vi "_Update Start Up Turbo.vi"(4 "error in (no error)":errorcluster) -> (0 "error Out":errorcluster, 2 "Next InstrState":T1, 3 "Cancel":bool)   [LabVIEW 2012]
uses:
  Type/_RT Instrument State.ctl
  Type/_LCD Line1 Msg.ctl
  Type/_LCD Line2 Msg.ctl
  Type/_Pump Parameter.ctl
  Type/_RW Status.ctl
  Type/_LED States.ctl
  _RT Global.vi
  <vilib>/Utility/error.llb/Error Cluster From Error Code.vi
  <vilib>/rvi/errors/niLvFpgaAdjustHostInterfaceError.vi
  <vilib>/rvi/interface/nirviReadWriteControl/nirviReadWriteControl.xnode
  FPGA Bitfiles/FPGA9602.lvbitx
  NiFpgaLv.dll
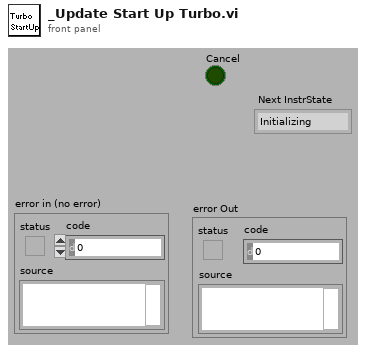
[diagram p1: front panel]
types:
  T1 = typedef "_RT Instrument State.ctl" = enum16{"Initializing", "Mass Spectrometer is Off", "Starting Up", "Turning Power Off", "Going to Standby", "Roughing Pump Ready", "Turning Turbo Off", "Turbo Startup", "Turbopump Ready", "Checking Vacuum", "Going to Ready", "Ready", "Running", "Source Standby", "Lost Communication", "Shutting Down", "Fault", "24V Standby", "Go to 24V Standby", "Turbopump Ready-Waiting"}
  T2 = typedef "_Pump Parameter.ctl" = enum16{"Turn Pump Motor On", "Turn Pump Motor Off", "Read Pump Oil Deficiency", "Read Rotation Switch Point Attained", "Read Ele. Drive Over Temperature", "Read Pump Over Temperature", "Read Set Rotation Speed Attained", "Read Turbopump Accelerates", "Read Actual Rotation Speed in Hz", "Read Motor Current in A", "Read Operating Hours in h", "Read Motor Voltage in V", "Read Motor Power in W", "Set Rotation Speed Switchpoint in %", "Clear Error", "Read Error Code", "Read Bearing Temperature", "Read Hardware Version", "Read Firmware Version", "Read Operating Hours (Drive)", "Read Rotational Speed (rpm)", "Read Power Stage Temperature", "Read Electronics Temperature", "Read Upper Pump Temperature", "Read Motor Temperature", "Read Error Code History, 1", "Read Error Code History, 2", "Read Error Code History, 3", "Read Error Code History, 4", "Read Error Code History, 5", "Read Error Code History, 6", "Read Error Code History, 7", "Read Error Code History, 8", "Read Error Code History, 9", "Read Error Code History, 10"}
  T3 = typedef "_RW Status.ctl" = enum8{"Done", "Do Read", "Do Write", "Set Latch1", "Set Latch2", "Set Latch3", "Set Latch4", "RP ON", "EL ON", "Serial Send", "Set LC Out", "Get LC In", "Read VAC", "Table Test", "Get Interlock", "Do Read2", "Do Write2"}
  T4 = typedef "_LED States.ctl" = enum8{"Idle", "Solid B", "Solid R", "Solid P", "Off B", "Off R", "Off P", "Off BRP", "Off RP", "Flash R&P", "Flash P"}
  T5 = typedef "_LCD Line2 Msg.ctl" = u16
  T6 = typedef "_LCD Line1 Msg.ctl" = u16
  T7 = typedef "_RT Startup Options.ctl" = cluster{"Door":bool, "Curtain":bool, "Pressure":bool, "Turbo":bool, "SysPoll":bool, "GasFlag":bool}
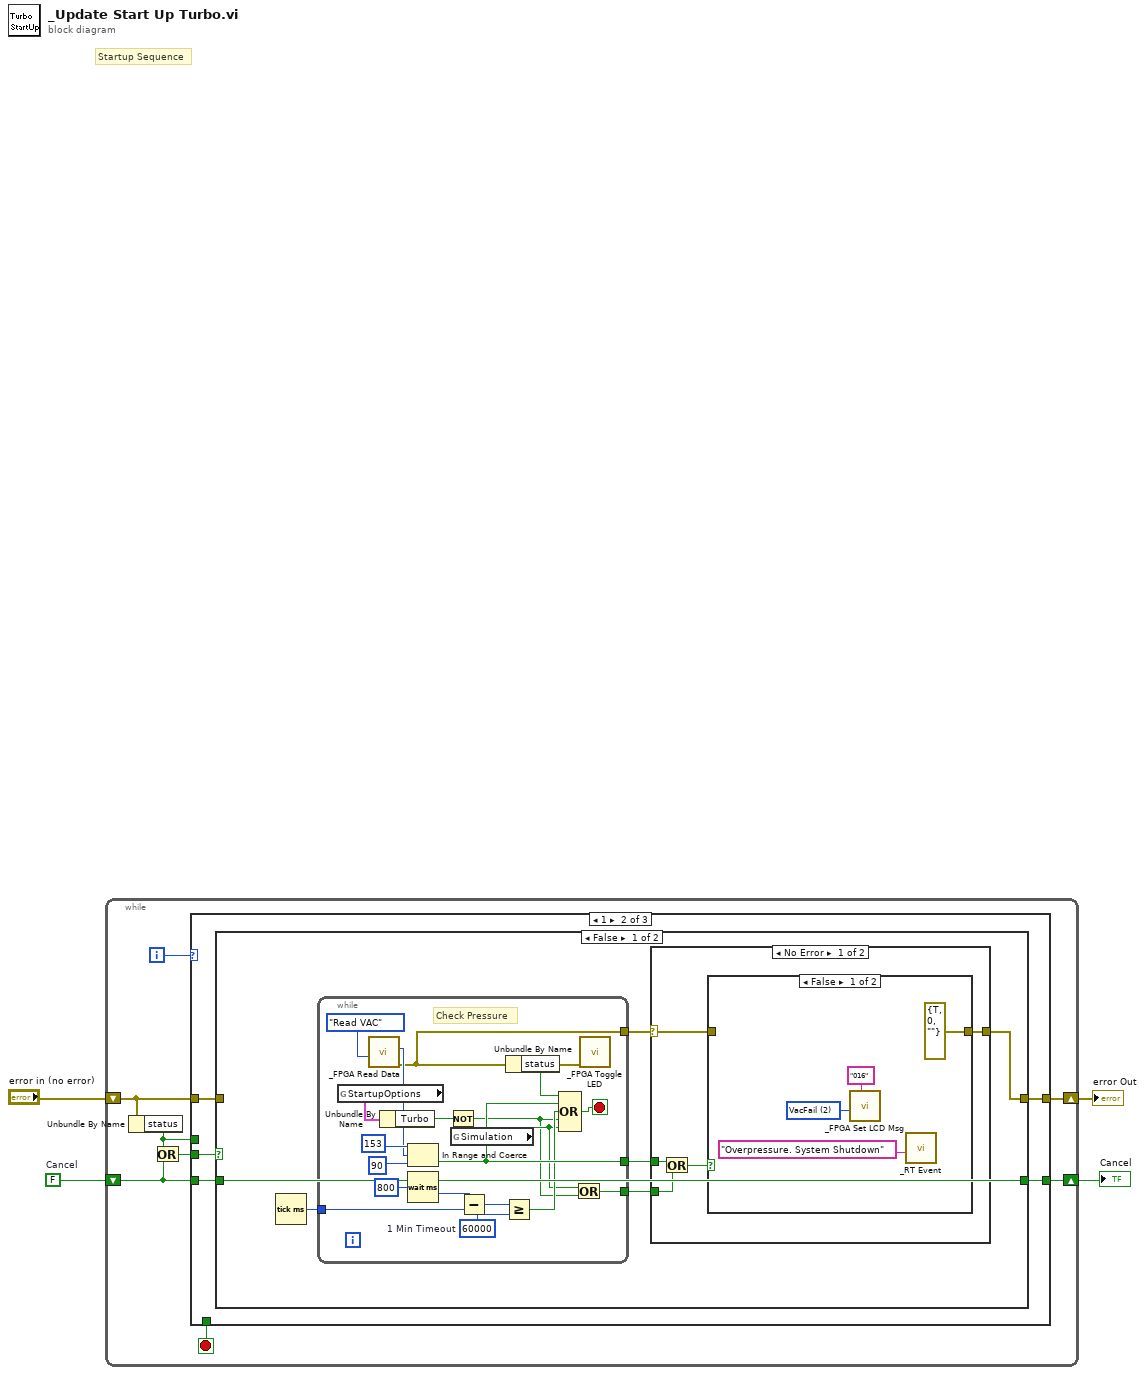
[diagram p0: block diagram]
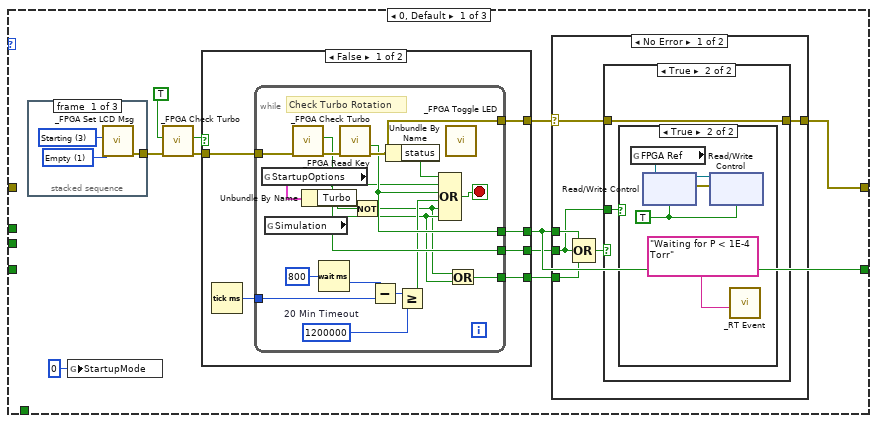
[diagram p2: hidden frame]
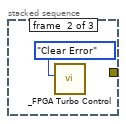
[diagram p3: hidden frame]
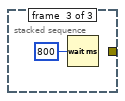
[diagram p4: hidden frame]
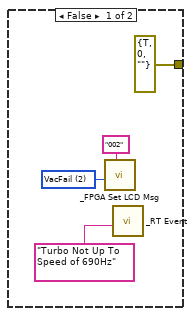
[diagram p6: hidden frame]
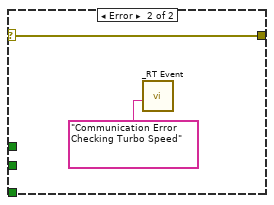
[diagram p8: hidden frame]
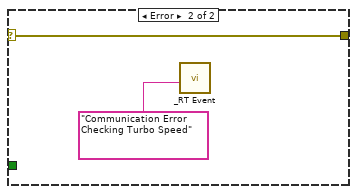
[diagram p10: hidden frame]
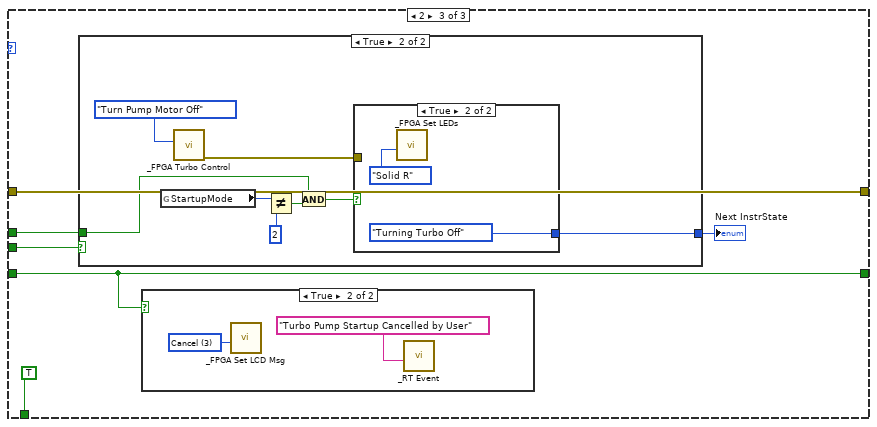
[diagram p12: hidden frame]
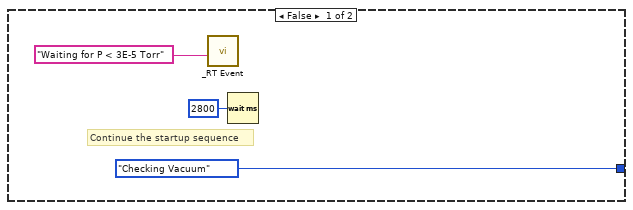
[diagram p13: hidden frame]
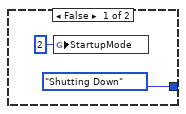
[diagram p14: hidden frame]
diagram:
  w3 = FALSE  # Cancel
  # "Startup Sequence"
  n1 = while {
    shift-right: [w8] -> w2
    shift-left: "error in (no error)" -> [w10]
    shift-right: [w7] -> w1
    shift-left: w3 -> [w9]
    i -> [w12]
    stop <- w6 stop-if-true
    n2 = Unbundle By Name(w10) -> ("status"=w5:bool)
    n3 = Or(x=w5, y=w9) -> (x .or. y?=w11:bool)
    n4 = case shown="1" w12 {
      tunnel: w11 -> [_ w75 w119]
      tunnel: w10 -> [_ w74 w121]
      tunnel: w9 -> [_ w73 w120]
      tunnel: [w22 w77 w121] -> w8
      tunnel: [w21 w76 w120] -> w7
      tunnel: [_ _ TRUE] -> w6
      tunnel: w5 -> [_ _ w117]
      frame 0, Default {
        n5 = stacked-sequence {
          tunnel: [w23 _ _] -> w13
          frame #0 {
            w24 = T5 1 items=["Same", "Empty", "VacFail", "Cancel", "CheckGas", "EleFail", "Probe1Fail", "Probe2Fail", "HeaterFail", "DoorOpen", "CheckComm", "PressStart", "StartRP"] ("Line2Msg (same)")
            w25 = T6 3 items=["Same", "Empty", "Connected", "Starting", "Stopping", "Action", "On", "Service", "Call", "Acquiring", "Source"] ("Line1Msg (same)")
            n6 = call "_FPGA Set LCD Msg.vi"("Line2Msg (same)"=w24, "Line1Msg (same)"=w25) -> ("error out"=w23:errorcluster)  [unwired: 5 in, 2 out]
          }
          frame #1 {
            n7 = call "_FPGA Turbo Control.vi"("Command"=_Pump_Parameter."Clear Error") -> ()  [unwired: 3 in, 6 out]
          }
          frame #2 {
            n8 = Wait (ms)(milliseconds to wait=u32 800) -> ()  [unwired: 1 out]
          }
        }
        n9 = global write "_RT Global.vi" "StartupMode"(u8 0 ("StartupMode")) -> ()
        n10 = call "_FPGA Check Turbo.vi"("error in"=w13, "CheckNow (F)"=TRUE) -> ("error out"=w18:errorcluster, "SpeedOK"=w16:bool)  [unwired: 1 in, 3 out]
        n11 = case shown="False" w16 {
          selector: w16 -> [_ w52]
          tunnel: [w33 _] -> w21
          tunnel: [w32 w53] -> w20
          tunnel: [w31 w52] -> w19
          tunnel: w18 -> [w29 w53]
          tunnel: [w28 _] -> w14
          frame False {
            n12 = Tick Count (ms)() -> (millisecond timer value=w30:u32)
            n13 = while {
              tunnel: w29 -> [w42]
              tunnel: [w48] -> w32
              tunnel: [w47] -> w33
              tunnel: w30 -> [w43]
              tunnel: [w40] -> w31
              tunnel: [w37] -> w28
              stop <- w51 stop-if-true
              w46 = u32 1200000  # 20 Min Timeout
              # "Check Turbo Rotation"
              n14 = global read "_RT Global.vi" "StartupOptions"() -> (w36:T7)
              n15 = global read "_RT Global.vi" "Simulation"() -> (w38:bool)
              n16 = call "_FPGA Check Turbo.vi"("error in"=w42) -> ("error out"=w41:errorcluster, "SpeedOK"=w40:bool)  [unwired: 1 in, 4 out]
              n17 = Unbundle By Name(w36) -> ("Turbo"=w35:bool)
              n18 = Wait (ms)(milliseconds to wait=u32 800) -> (millisecond timer value=w44:u32)
              n19 = call "_FPGA Read Key.vi"("error in (no error)"=w41) -> ("error out"=w48:errorcluster, "Key Pressed"=w47:bool)  [unwired: 4 in, 2 out]
              n20 = Not(x=w35) -> (.not. x?=w34:bool)
              n21 = Subtract(x=w44, y=w43) -> (x-y=w45:u32)
              n22 = Unbundle By Name(w48) -> ("status"=w50:bool)
              n23 = Greater Or Equal?(x=w45, y=w46) -> (x >= y?=w39:bool)
              n24 = Compound Arithmetic op=OR(w50, w40, w47, w39, w34, w38) -> (w51:bool)
              n25 = call "_FPGA Toggle LED.vi"() -> ()  [unwired: 5 in, 4 out]
              n26 = Or(x=w34, y=w38) -> (x .or. y?=w37:bool)
            }
          }
          frame True {
          }
        }
        n27 = case shown="No Error" w20 {
          selector: w20 -> [w59 w72]
          tunnel: w19 -> [w55 _]
          tunnel: [w58 w72] -> w22
          tunnel: w21 -> [w56 _]
          tunnel: w14 -> [w54 _]
          frame No Error {
            n28 = Compound Arithmetic op=OR(w56, w55, w54) -> (w57:bool)
            n29 = case shown="True" w57 {
              tunnel: [errorcluster {"status"=TRUE, "code"=0, "source"=""} ("error IO") w65] -> w58
              tunnel: w59 -> [_ w65]
              tunnel: w55 -> [_ w64]
              frame False {
                w61 = T5 2 items=["Same", "Empty", "VacFail", "Cancel", "CheckGas", "EleFail", "Probe1Fail", "Probe2Fail", "HeaterFail", "DoorOpen", "CheckComm", "PressStart", "StartRP"] ("Line2Msg (same)")
                n30 = call "_FPGA Set LCD Msg.vi"("ErrNum"="002", "Line2Msg (same)"=w61) -> ()  [unwired: 4 in, 4 out]
                n31 = call "_RT Event.vi"("Event"="Turbo Not Up To      Speed of 690Hz" ("Command")) -> ()  [unwired: 2 in, 5 out]
              }
              frame True {
                n32 = case shown="True" w64 {
                  frame False {
                  }
                  frame True {
                    w70 = TRUE
                    n33 = global read "_RT Global.vi" "FPGA Ref"() -> (w66:refnum<k20>)
                    n34 = xnode "Read/Write Control"("FPGA VI Reference In"=w66, "FilaB"=w70) -> ("FPGA VI Reference Out"=w68:refnum<k20>, "error out"=w69:errorcluster)  [unwired: 1 in]
                    n35 = xnode "Read/Write Control"("FPGA VI Reference In"=w68, "error in"=w69, "FilaC"=w70) -> ()  [unwired: 2 out]
                    n36 = call "_RT Event.vi"("Event"="Waiting for P < 1E-4 Torr" ("Command")) -> ()  [unwired: 2 in, 5 out]
                  }
                }
              }
            }
          }
          frame Error {
            n37 = call "_RT Event.vi"("Event"="Communication Error Checking Turbo Speed") -> ()  [unwired: 2 in, 5 out]
          }
        }
      }
      frame 1 {
        n38 = case shown="False" w75 {
          tunnel: [w79 w115] -> w76
          tunnel: [w81 w116] -> w77
          tunnel: w74 -> [_ w116]
          tunnel: w73 -> [w79 w115]
          frame False {
            n39 = Tick Count (ms)() -> (millisecond timer value=w80:u32)
            n40 = while {
              tunnel: [w84] -> w83
              tunnel: w80 -> [w98]
              tunnel: [w96] -> w82
              tunnel: [w88] -> w78
              stop <- w102 stop-if-true
              w92 = u32 60000  # 1 Min Timeout
              # "Check Pressure"
              n41 = global read "_RT Global.vi" "StartupOptions"() -> (w87:T7)
              n42 = call "_FPGA Read Data.vi"("Read Mode (Do Read)"=_RW_Status."Read VAC" ("R/W Status")) -> ("error out"=w84:errorcluster, "Data"=w93:u32)  [unwired: 4 in, 1 out]
              n43 = Unbundle By Name(w87) -> ("Turbo"=w86:bool)
              n44 = In Range and Coerce(upper limit=u32 153, x=w93, lower limit=u32 90 ("y")) -> (In Range?=w96:bool)  [unwired: 1 out]
              n45 = Wait (ms)(milliseconds to wait=u32 800) -> (millisecond timer value=w99:u32)
              n46 = Not(x=w86) -> (.not. x?=w85:bool)
              n47 = global read "_RT Global.vi" "Simulation"() -> (w89:bool)
              n48 = Subtract(x=w99, y=w98) -> (x-y=w91:u32)
              n49 = Greater Or Equal?(x=w91, y=w92) -> (x >= y?=w90:bool)
              n50 = Unbundle By Name(w84) -> ("status"=w101:bool)
              n51 = Compound Arithmetic op=OR(w101, w96, w90, w85, w89) -> (w102:bool)
              n52 = Or(x=w89, y=w85) -> (x .or. y?=w88:bool)
              n53 = call "_FPGA Toggle LED.vi"("error in (no error)"=w84) -> ()  [unwired: 4 in, 4 out]
            }
            n54 = case shown="No Error" w83 {
              selector: w83 -> [w107 w114]
              tunnel: w82 -> [w103 _]
              tunnel: [w106 w114] -> w81
              tunnel: w78 -> [w104 _]
              frame No Error {
                n55 = Or(x=w103, y=w104) -> (x .or. y?=w105:bool)
                n56 = case shown="False" w105 {
                  tunnel: [errorcluster {"status"=TRUE, "code"=0, "source"=""} ("error IO") w112] -> w106
                  tunnel: w107 -> [_ w112]
                  frame False {
                    w109 = T5 2 items=["Same", "Empty", "VacFail", "Cancel", "CheckGas", "EleFail", "Probe1Fail", "Probe2Fail", "HeaterFail", "DoorOpen", "CheckComm", "PressStart", "StartRP"] ("Line2Msg (same)")
                    n57 = call "_FPGA Set LCD Msg.vi"("ErrNum"="016", "Line2Msg (same)"=w109) -> ()  [unwired: 4 in, 4 out]
                    n58 = call "_RT Event.vi"("Event"="Overpressure. System Shutdown" ("Command")) -> ()  [unwired: 2 in, 5 out]
                  }
                  frame True {
                  }
                }
              }
              frame Error {
                n59 = call "_RT Event.vi"("Event"="Communication Error Checking Turbo Speed") -> ()  [unwired: 2 in, 5 out]
              }
            }
          }
          frame True {
          }
        }
      }
      frame 2 {
        n60 = case shown="True" w119 {
          tunnel: [_RT_Instrument_State."Checking Vacuum" ("Next InstrState") w132] -> w118
          tunnel: w117 -> [_ w128]
          frame False {
            # "Continue the startup sequence"
            n61 = call "_RT Event.vi"("Event"="Waiting for P < 3E-5 Torr" ("Command")) -> ()  [unwired: 2 in, 5 out]
            n62 = Wait (ms)(milliseconds to wait=u32 2800) -> ()  [unwired: 1 out]
          }
          frame True {
            n63 = global read "_RT Global.vi" "StartupMode"() -> (w131:u8)
            n64 = call "_FPGA Turbo Control.vi"("Command"=_Pump_Parameter."Turn Pump Motor Off") -> ("error out"=w126:errorcluster)  [unwired: 3 in, 5 out]
            n65 = Not Equal?(x=w131, y=u8 2) -> (x != y?=w129:bool)
            n66 = And(x=w128, y=w129) -> (x .and. y?=w127:bool)
            n67 = case shown="True" w127 {
              tunnel: [_RT_Instrument_State."Shutting Down" ("Next InstrState") _RT_Instrument_State."Turning Turbo Off" ("Next InstrState")] -> w132
              tunnel: w126 -> [_ _]
              frame False {
                n68 = global write "_RT Global.vi" "StartupMode"(u8 2 ("StartupMode")) -> ()
              }
              frame True {
                n69 = call "_FPGA Set LEDs.vi"("LED Command"=_LED_States."Solid R") -> ()  [unwired: 3 in, 4 out]
              }
            }
          }
        }
        "Next InstrState" <- w118
        n70 = case shown="True" w120 {
          frame False {
          }
          frame True {
            w139 = T5 3 items=["Same", "Empty", "VacFail", "Cancel", "CheckGas", "EleFail", "Probe1Fail", "Probe2Fail", "HeaterFail", "DoorOpen", "CheckComm", "PressStart", "StartRP"] ("Line2Msg (same)")
            n71 = call "_FPGA Set LCD Msg.vi"("Line2Msg (same)"=w139) -> ()  [unwired: 6 in, 3 out]
            n72 = call "_RT Event.vi"("Event"="Turbo Pump Startup Cancelled by User" ("Command")) -> ()  [unwired: 2 in, 5 out]
          }
        }
      }
    }
  }
  "error Out" <- w2
  "Cancel" <- w1
